vi "set column.vi"(0 "VISA in":refnum<visa-resource-name>, 1 "Location Cluster in":T1, 2 "set column":i32, 5 "error in":errorcluster) -> (14 "VISA out":refnum<visa-resource-name>, 15 "Location Cluster out":T1, 19 "error out":errorcluster)   [LabVIEW 2018]
uses:
  location cluster.ctl
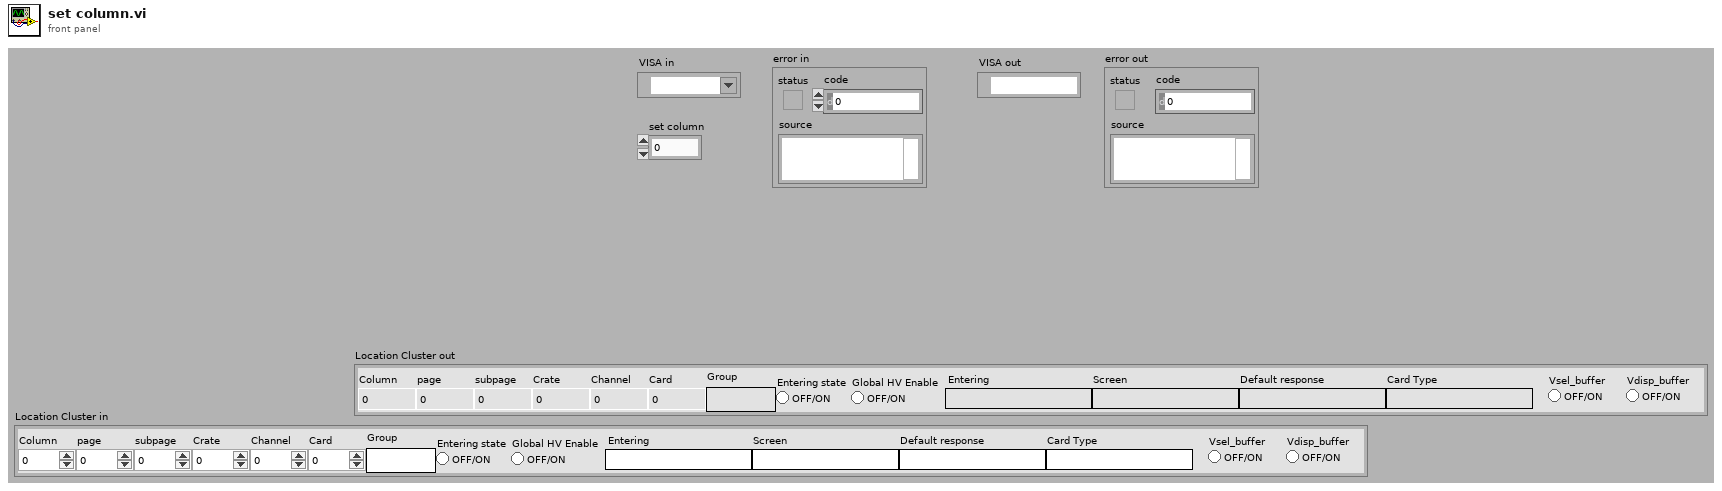
[diagram p1: front panel]
types:
  T1 = typedef "location cluster.ctl" = cluster{"Column":i32, "Card Type":string, "Channel":i32, "Card":i32, "Default response":string, "Entering":string, "Entering state":bool, "subpage":i32, "page":i32, "Crate":i32, "Screen":string, "Group":string, "Global HV Enable":bool, "Vsel_buffer":bool, "Vdisp_buffer":bool}
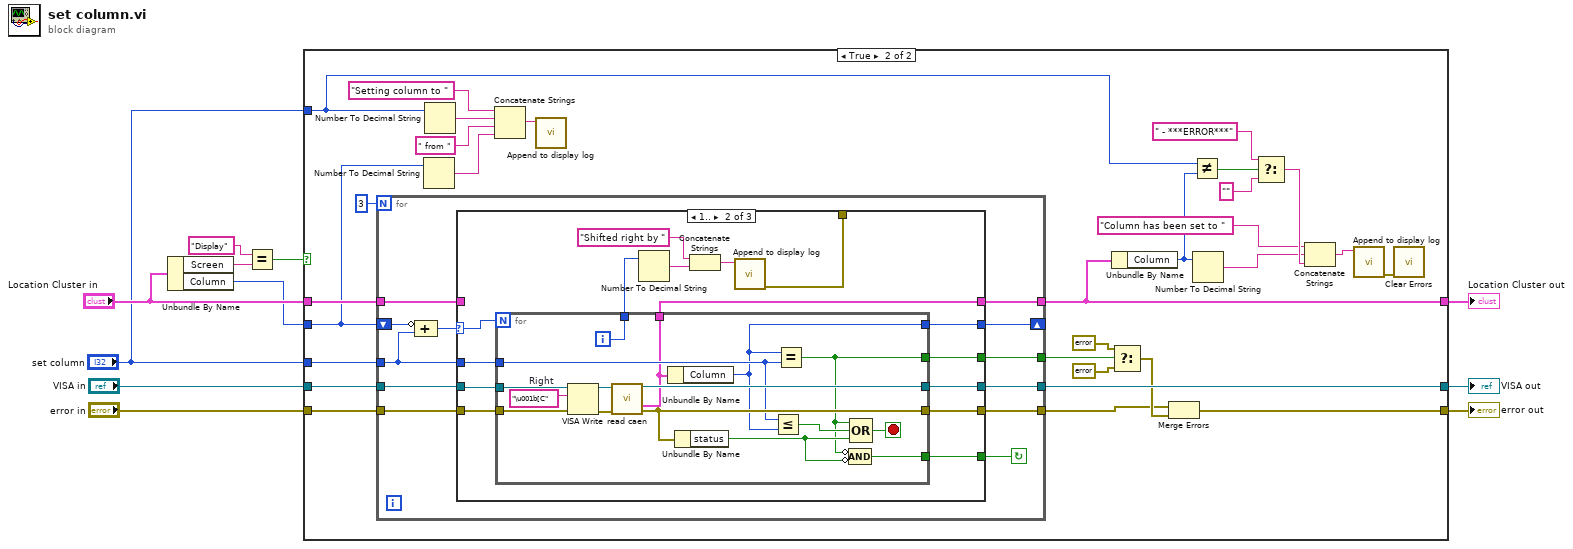
[diagram p0: block diagram]
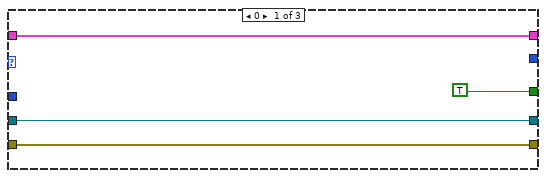
[diagram p3: hidden frame]
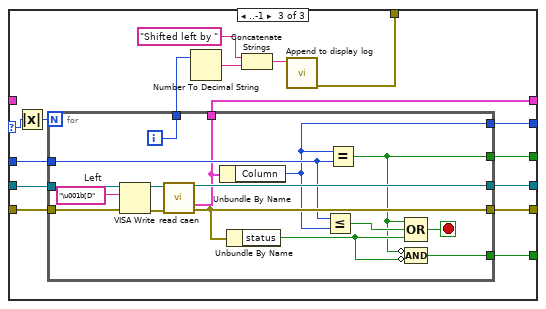
[diagram p4: hidden frame]
diagram:
  n1 = Unbundle By Name("Location Cluster in") -> ("Screen"=w6:string, "Column"=w3:i32)
  n2 = Equal?(x="Display", y=w6) -> (x = y?=w4:bool)
  n3 = case shown="True" w4 {
    tunnel: [w12 w35] -> w11
    tunnel: [w13 w43] -> w10
    tunnel: [w14 w16] -> w1
    tunnel: "set column" -> [_ w42]
    tunnel: "error in" -> [w12 w41]
    tunnel: "VISA in" -> [w13 w40]
    tunnel: "Location Cluster in" -> [w14 w39]
    tunnel: w3 -> [_ w26]
    tunnel: "set column" -> [_ w15]
    frame False {
    }
    frame True {
      n4 = for {
        N: 3 -> [_]
        shift-right: [w47] -> _
        shift-left: w26 -> [w48]
        tunnel: w40 -> [w51]
        tunnel: [w55] -> w43
        tunnel: w41 -> [w52]
        tunnel: [w46] -> w36
        tunnel: w42 -> [w53]
        tunnel: w39 -> [w49]
        tunnel: [w54] -> w16
        tunnel: [w44] -> w34
        stop <- w45 continue-if-true
        n5 = Compound Arithmetic op=ADD(invert w48, w53) -> (w50:i32)
        n6 = case shown="1.." w50 {
          selector: w50 -> [_ w60 w92]
          tunnel: [w59 w63 w95] -> w55
          tunnel: w51 -> [w59 w74 w106]
          tunnel: w52 -> [w58 w73 w105]
          tunnel: [w58 w64 w96] -> w46
          tunnel: [w57 w65 w97] -> w54
          tunnel: w49 -> [w57 _ _]
          tunnel: w53 -> [_ w72 w104]
          tunnel: [_ w67 w99] -> _
          tunnel: [_ w66 w98] -> w47
          tunnel: [TRUE w62 w94] -> w44
          tunnel: [_ w61 w93] -> w45
          frame 0 {
          }
          frame 1.. {
            n7 = for {
              N: w60 -> [_]
              tunnel: w74 -> [w90]
              tunnel: w73 -> [w89]
              tunnel: [w86] -> w63
              tunnel: [w85] -> w64
              tunnel: w72 -> [w82]
              tunnel: [w75] -> w62
              tunnel: [w81] -> w68
              tunnel: [w80] -> w66
              tunnel: [w79] -> w65
              tunnel: [w76] -> w61
              i -> [w81]
              stop <- w84 stop-if-true
              w83 = "\u001b[C"  # Right
              n8 = VISA Write(VISA resource name=w90, write buffer=w83, error in (no error)=w89) -> (VISA resource name out=w88:refnum<visa-resource-name>, error out=w87:errorcluster)  [unwired: 1 out]
              n9 = call "read caen.vi"("VISA in"=w88, "error in"=w87) -> ("VISA out"=w86:refnum<visa-resource-name>, "Location Cluster"=w79:T1, "error out"=w85:errorcluster)  [unwired: 8 in, 3 out]
              n10 = Unbundle By Name(w79) -> ("Column"=w80:i32)
              n11 = Unbundle By Name(w85) -> ("status"=w77:bool)
              n12 = Less Or Equal?(x=w82, y=w80) -> (x <= y?=w78:bool)
              n13 = Equal?(x=w80, y=w82) -> (x = y?=w75:bool)
              n14 = Compound Arithmetic op=AND(invert w75, invert w77) -> (w76:bool)
              n15 = Compound Arithmetic op=OR(w75, w78, w77) -> (w84:bool)
            }
            n16 = Number To Decimal String(number=w68) -> (decimal integer string=w69:string)  [unwired: 1 in]
            n17 = Concatenate Strings("Shifted right by " ("string"), w69) -> (w70:string)
            n18 = call "Append to display log.vi"("string"=w70) -> ("error out"=w67:errorcluster)  [unwired: 10 in]
          }
          frame ..-1 {
            n19 = Absolute Value(x=w92) -> (abs(x)=w91:i32)
            n20 = for {
              N: w91 -> [_]
              tunnel: w106 -> [w122]
              tunnel: w105 -> [w121]
              tunnel: [w118] -> w95
              tunnel: [w117] -> w96
              tunnel: w104 -> [w115]
              tunnel: [w107] -> w94
              tunnel: [w114] -> w100
              tunnel: [w113] -> w98
              tunnel: [w112] -> w97
              tunnel: [w108] -> w93
              i -> [w114]
              stop <- w116 stop-if-true
              w111 = "\u001b[D"  # Left
              n21 = VISA Write(VISA resource name=w122, write buffer=w111, error in (no error)=w121) -> (VISA resource name out=w120:refnum<visa-resource-name>, error out=w119:errorcluster)  [unwired: 1 out]
              n22 = call "read caen.vi"("VISA in"=w120, "error in"=w119) -> ("VISA out"=w118:refnum<visa-resource-name>, "Location Cluster"=w112:T1, "error out"=w117:errorcluster)  [unwired: 8 in, 3 out]
              n23 = Unbundle By Name(w112) -> ("Column"=w113:i32)
              n24 = Unbundle By Name(w117) -> ("status"=w109:bool)
              n25 = Less Or Equal?(x=w115, y=w113) -> (x <= y?=w110:bool)
              n26 = Equal?(x=w113, y=w115) -> (x = y?=w107:bool)
              n27 = Compound Arithmetic op=OR(w107, w110, w109) -> (w116:bool)
              n28 = Compound Arithmetic op=AND(invert w107, invert w109) -> (w108:bool)
            }
            n29 = Number To Decimal String(number=w100) -> (decimal integer string=w101:string)  [unwired: 1 in]
            n30 = Concatenate Strings("Shifted left by " ("string"), w101) -> (w102:string)
            n31 = call "Append to display log.vi"("string"=w102) -> ("error out"=w99:errorcluster)  [unwired: 10 in]
          }
        }
      }
      n32 = Number To Decimal String(number=w26) -> (decimal integer string=w31:string)  [unwired: 1 in]
      n33 = Number To Decimal String(number=w15) -> (decimal integer string=w28:string)  [unwired: 1 in]
      n34 = Concatenate Strings("Setting column to " ("string"), w28, " from " ("string"), w31) -> (w30:string)
      n35 = call "Append to display log.vi"("string"=w30) -> ()  [unwired: 10 in, 1 out]
      n36 = Unbundle By Name(w16) -> ("Column"=w24:i32)
      n37 = Select(t=errorcluster {"status"=FALSE, "code"=0, "source"=""} ("f"), s=w34, f=errorcluster {"status"=TRUE, "code"=0, "source"="Column num inaccessible!"} ("input cluster")) -> (s? t:f=w37:errorcluster)
      n38 = Merge Errors(w36, w37) -> (w35:errorcluster)
      n39 = Not Equal?(x=w15, y=w24) -> (x != y?=w21:bool)
      n40 = Number To Decimal String(number=w24) -> (decimal integer string=w20:string)  [unwired: 1 in]
      n41 = Select(t=" - ***ERROR***" ("string"), s=w21, f="" ("string")) -> (s? t:f=w25:string)
      n42 = Concatenate Strings("Column has been set to " ("string"), w20, w25) -> (w19:string)
      n43 = call "Append to display log.vi"("string"=w19) -> ("error out"=w17:errorcluster)  [unwired: 10 in]
      n44 = call <vilib>:"Clear Errors.vi"("error in (no error)"=w17) -> ()  [unwired: 5 in, 2 out]
    }
  }
  "error out" <- w11
  "VISA out" <- w10
  "Location Cluster out" <- w1
